vi "Error Internal Library Implementation Error.vi"() -> (0 "Error Code":i32)   [LabVIEW 2020, in "serenial.io-ase.lvlib" / "ase.lvclass"]
doc: "Error code constant"
uses:
  ase.lvclass
  ase.lvclass/ase.ctl
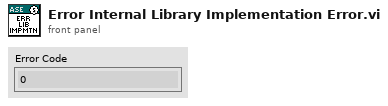
[diagram p1: front panel]
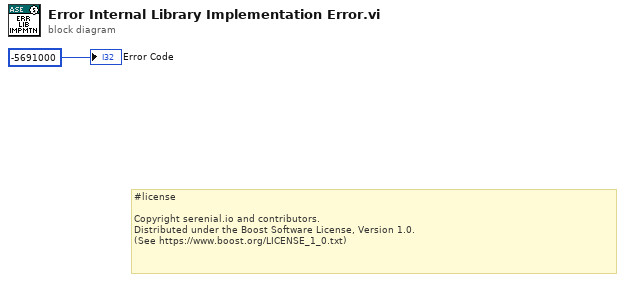
[diagram p0: block diagram]
diagram:
  # "#license\n\nCopyright serenial.io and contributors.\nDistributed under the Boost Software License, Version 1.0.\n(See https://www.boost.org/LICENSE_1_0.txt)"
  "Error Code" <- -5691000 ("error code (0)")
